vi "create MonthlyExpense.vi"(5 "Target Account":string, 7 "Source Account":string, 8 "error in (no error)":errorcluster, 9 "Amount":dbl, 10 "Name":string, 11 "MonthlyExpense in":refnum<class "MonthlyExpense.lvclass">) -> (0 "error out":errorcluster, 3 "MonthlyExpense out":refnum<class "MonthlyExpense.lvclass">)   [LabVIEW 2020, in "MonthlyExpense.lvclass"]
uses:
  MonthlyExpense.lvclass
  MonthlyExpense.lvclass/MonthlyExpense.ctl
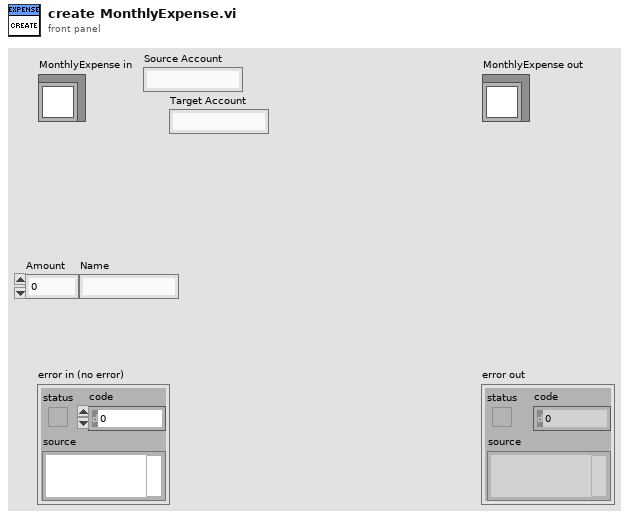
[diagram p1: front panel]
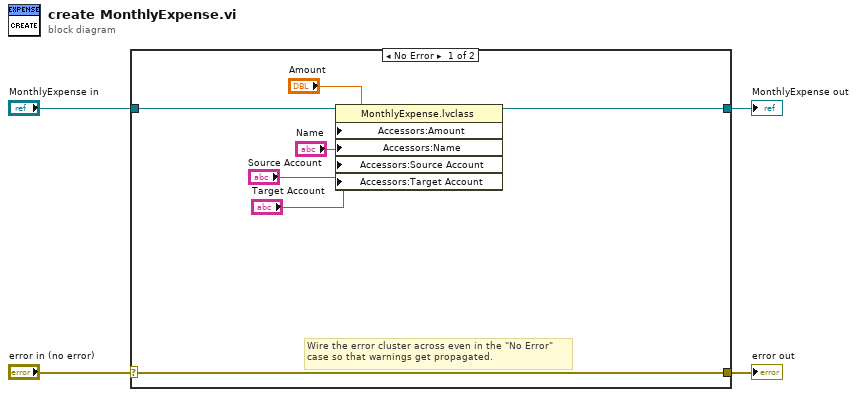
[diagram p0: block diagram]
diagram:
  n1 = case shown="No Error" "error in (no error)" {
    selector: "error in (no error)" -> [w10 w13]
    tunnel: [w10 w13] -> w3
    tunnel: [w9 w12] -> w1
    tunnel: "MonthlyExpense in" -> [w11 w12]
    frame No Error {
      # "Wire the error cluster across even in the \"No Error\"\ncase so that warnings get propagated."
      n2 = property class="MonthlyExpense.lvclass"(reference=w11, "Accessors:Amount"="Amount", "Accessors:Name"="Name", "Accessors:Source Account"="Source Account", "Accessors:Target Account"="Target Account") -> (reference out=w9:refnum<class "MonthlyExpense.lvclass">)  [unwired: 1 in, 1 out]
    }
    frame Error {
    }
  }
  "error out" <- w3
  "MonthlyExpense out" <- w1
